vi "Add Test Suite.vi"(10 "Test Suite to add":refnum<class "LUnit Test Suite.lvclass">, 11 "Test Suite In":refnum<class "LUnit Test Suite.lvclass">) -> (3 "Test Suite Out":refnum<class "LUnit Test Suite.lvclass">)   [LabVIEW 2020, in "LUnit Test Suite.lvclass"]
uses:
  LUnit Test Suite.lvclass
  LUnit Test Suite.lvclass/LUnit Test Suite.ctl
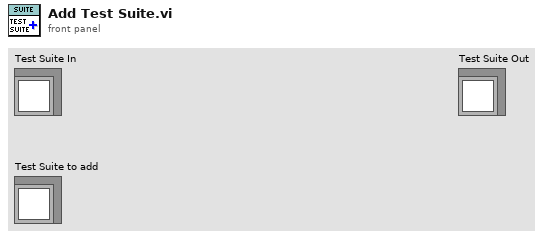
[diagram p1: front panel]
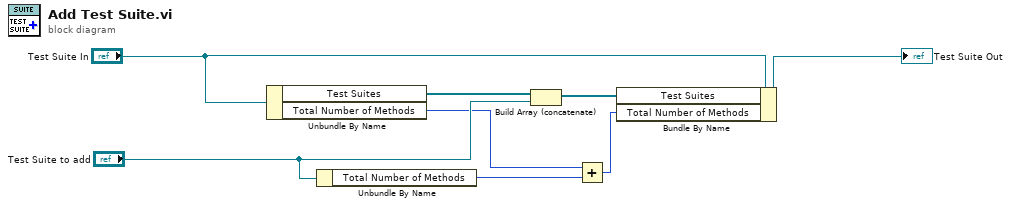
[diagram p0: block diagram]
diagram:
  n1 = Unbundle By Name("Test Suite In") -> ("Test Suites"=w7:refnum<class>[], "Total Number of Methods"=w3:i32)
  n2 = Unbundle By Name("Test Suite to add") -> ("Total Number of Methods"=w2:i32)
  n3 = Build Array (concatenate)(w7, "Test Suite to add") -> (w5:refnum<class>[])
  n4 = Add(x=w3, y=w2) -> (x+y=w1:i32)
  n5 = Bundle By Name(cluster="Test Suite In", "Test Suites"=w5, "Total Number of Methods"=w1) -> (→"Test Suite Out":refnum<class "LUnit Test Suite.lvclass">)
